vi "Wrist main.vi"() -> ()   [LabVIEW 2018]
uses:
  <vilib>/Rock Robotics/WPI/ThirdParty/Phoenix-LabVIEW/Motor Controller/Controls/CTRE_Phoenix_MotorControl_FeedbackDevice.ctl
  <vilib>/Rock Robotics/WPI/ThirdParty/Phoenix-LabVIEW/Motor Controller/Controls/CTRE_Phoenix_MotorControl_ControlMode.ctl
  <vilib>/Rock Robotics/WPI/ThirdParty/Phoenix-LabVIEW/Motor Controller/Get/CTRE_Phoenix_MotorController_GetSelectedSensorData.vi
panel:
  in  "reset pos":bool
  out "Wrist at home":bool
  in  "Disable?":bool
  in  "Wrist Selector":enum16{"Motion Magic", "Manual", "Disable"}(ring)
  in  "Output":dbl(slide) scale=-1.0..1.0
  in  "Setpoint":dbl
  in  "PIDF":T1={"P"=1.5, "I"=0.0005, "D"=0.0, "F"=0.0, "I zone"=0.0}
  out "Velocity (Raw Sensor Units per 100 ms)":i32
  out "Position (Raw Sensor Units)":i32
  in  "Acceleration":i32
  in  "Cruise Velocity":i32
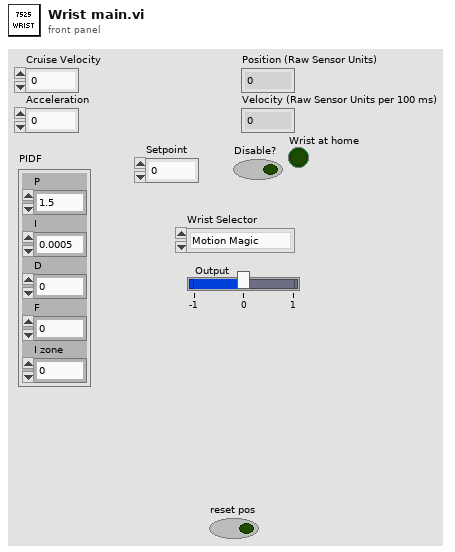
[diagram p1: front panel]
types:
  T1 = cluster{"P":dbl, "I":dbl, "D":dbl, "F":dbl, "I zone":dbl}
  T2 = typedef "CTRE_Phoenix_MotorControl_FeedbackDevice.ctl" = i8
  T3 = typedef "WPI_MotorControlDeviceRef.ctl" = cluster{"DeviceStatus":errorcluster, "Type":T4, "PWM":cluster{"PWM Channel":T5, "DeadBand":T6}, "CAN":cluster{"Device Number":u8, "SetOutput VI Ref":variant, "GetOutput VI Ref":variant, "Enable VI Ref":variant, "Disable VI Ref":variant, "Data":variant}, "Invert":bool, "DIO PWM":cluster{"PWM \"Enable\" Channel":T5, "DIOChannel":T7, "PWM Rate":dbl}}
  T4 = typedef "WPI_MotorControlType.ctl" = enum16{"PWM", "CAN", "DIO PWM"}
  T5 = typedef "FPGA_DIOPWMChannel.ctl" = enum8{"PWM 0", "PWM 1", "PWM 2", "PWM 3", "PWM 4", "PWM 5", "PWM 6", "PWM 7", "PWM 8", "PWM 9", "PWM MXP 0", "PWM MXP 1", "PWM MXP 2", "PWM MXP 3", "PWM MXP 4", "PWM MXP 5", "PWM MXP 6", "PWM MXP 7", "PWM MXP 8", "PWM MXP 9", "Invalid"}
  T6 = typedef "WPI_PWMDeadband.ctl" = cluster{"Name":string, "maxPositivePwm":i32, "minPositivePwm":i32, "centerPwm":i32, "maxNegativePwm":i32, "minNegativePwm":i32, "angularRange":u16}
  T7 = typedef "FPGA_DIOChannel.ctl" = enum8{"DIO 0", "DIO 1", "DIO 2", "DIO 3", "DIO 4", "DIO 5", "DIO 6", "DIO 7", "DIO 8", "DIO 9", "DIO MXP 0", "DIO MXP 1", "DIO MXP 2", "DIO MXP 3", "DIO MXP 4", "DIO MXP 5", "DIO MXP 6", "DIO MXP 7", "DIO MXP 8", "DIO MXP 9", "DIO MXP 10", "DIO MXP 11", "DIO MXP 12", "DIO MXP 13", "DIO MXP 14", "DIO MXP 15", "SPI Port CS1", "SPI Port CS2", "SPI Port CS3", "SPI Port MISO", "SPI Port MOSI", "Invalid"}
  T8 = typedef "CTRE_Phoenix_MotorControl_ControlMode.ctl" = u16
  T9 = typedef "WPI_SwitchDevRef.ctl" = cluster{"DevStatus":errorcluster, "DIO Channel":T7, "CntIndex":T10, "Normally Closed":bool}
  T10 = typedef "FPGA_CounterCtrSystemIndex.ctl" = enum8{"Ctr 0", "Ctr 1", "Ctr 2", "Ctr 3", "Ctr 4", "Ctr 5", "Ctr 6", "Ctr 7", "Invalid"}
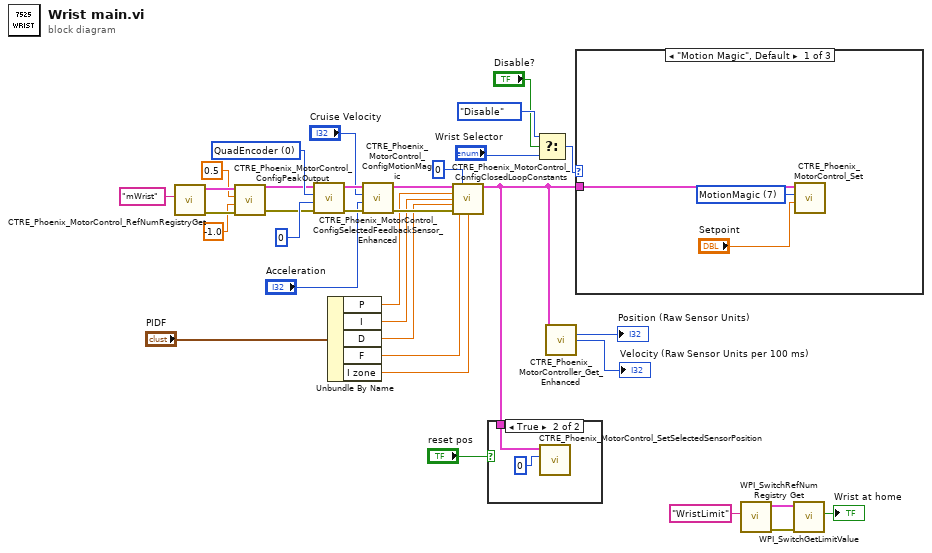
[diagram p0: block diagram]
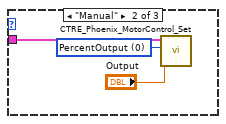
[diagram p3: hidden frame]
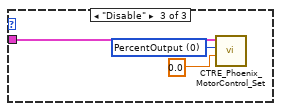
[diagram p4: hidden frame]
diagram:
  w29 = T2 0 items=["QuadEncoder"=0, "Analog"=2, "Tachometer"=4, "Pulse Width Encoded Position"=8, "Sensor Sum (S0 + S1)"=9, "Sensor Difference (D0 - D1)"=10, "Remote Source 0"=11, "Remote Source 1"=12, "Software Emulated"=15] ("Feedback Device")
  n1 = call <vilib>:"CTRE_Phoenix_MotorControl_RefNumRegistryGet.vi"("refnum name"="mWrist") -> ("error out"=w33:errorcluster, "PhoenixMotorControlDevRef"=w32:T3)  [unwired: 9 in]
  n2 = call <vilib>:"CTRE_Phoenix_MotorControl_ConfigPeakOutput.vi"("error in (no error)"=w33, "Reverse Peak Percent Output"=-1.0, "Forward Peak Percent Output"=0.5, "PhoenixMotorControlDevRef"=w32) -> ("error out"=w26:errorcluster, "PhoenixMotorControlDevRef"=w27:T3)  [unwired: 6 in]
  n3 = call <vilib>:"CTRE_Phoenix_MotorControl_ConfigSelectedFeedbackSensor_Enhanced.vi"("error in (no error)"=w26, "pidLoopIdx"=0, "Feedback Device"=w29, "PhoenixMotorControlDevRef"=w27) -> ("error out"=w25:errorcluster, "PhoenixMotorControlDevRef"=w24:T3)  [unwired: 6 in]
  n4 = Unbundle By Name("PIDF") -> ("P"=w15:dbl, "I"=w14:dbl, "D"=w13:dbl, "F"=w12:dbl, "I zone"=w11:dbl)
  n5 = call <vilib>:"CTRE_Phoenix_MotorControl_ConfigMotionMagic.vi"("error in (no error)"=w25, "Acceleration"="Acceleration", "Cruise Velocity"="Cruise Velocity", "PhoenixMotorControlDevRef"=w24) -> ("error out"=w18:errorcluster, "PhoenixMotorControlDevRef"=w19:T3)  [unwired: 6 in]
  n6 = call <vilib>:"CTRE_Phoenix_MotorControl_ConfigClosedLoopConstants.vi"("PhoenixMotorControlDevRef"=w19, "slotIdx"=0, "P"=w15, "I"=w14, "D"=w13, "error in (no error)"=w18, "F"=w12, "I Zone"=w11) -> ("PhoenixMotorControlDevRef"=w1:T3)  [unwired: 6 in, 1 out]
  n7 = case shown="True" "reset pos" {
    tunnel: w1 -> [_ w36]
    frame False {
    }
    frame True {
      n8 = call <vilib>:"CTRE_Phoenix_MotorControl_SetSelectedSensorPosition.vi"("New Sensor Position"=0, "PhoenixMotorControlDevRef"=w36) -> ()  [unwired: 8 in, 2 out]
    }
  }
  n9 = Select(t=enum16{"Motion Magic", "Manual", "Disable"}."Disable", s="Disable?", f="Wrist Selector") -> (s? t:f=w9:enum16{"Motion Magic", "Manual", "Disable"})
  n10 = call-poly <vilib>:"CTRE_Phoenix_MotorController_Get_Enhanced.vi"("PhoenixMotorControlDevRef"=w1) -> ("Position (Raw Sensor Units)"=→"Position (Raw Sensor Units)":i32, "Velocity (Raw Sensor Units per 100 ms)"=→"Velocity (Raw Sensor Units per 100 ms)":i32)  [unwired: 11 in, 2 out]
  n11 = case shown="\"Motion Magic\", Default" w9 {
    tunnel: w1 -> [w38 w42 w44]
    frame "Motion Magic", Default {
      w39 = T8 7 items=["PercentOutput"=0, "Position"=1, "Velocity"=2, "Current"=3, "Follower"=5, "MotionProfile"=6, "MotionMagic"=7, "MotionProfileArc"=10, "Disabled"=15] ("Control Mode")
      n12 = call <vilib>:"CTRE_Phoenix_MotorControl_Set.vi"("Output"="Setpoint", "Control Mode"=w39, "PhoenixMotorControlDevRef"=w38) -> ()  [unwired: 7 in, 2 out]
    }
    frame "Manual" {
      w41 = T8 0 items=["PercentOutput"=0, "Position"=1, "Velocity"=2, "Current"=3, "Follower"=5, "MotionProfile"=6, "MotionMagic"=7, "MotionProfileArc"=10, "Disabled"=15] ("Control Mode")
      n13 = call <vilib>:"CTRE_Phoenix_MotorControl_Set.vi"("Output"="Output", "Control Mode"=w41, "PhoenixMotorControlDevRef"=w42) -> ()  [unwired: 7 in, 2 out]
    }
    frame "Disable" {
      w45 = T8 0 items=["PercentOutput"=0, "Position"=1, "Velocity"=2, "Current"=3, "Follower"=5, "MotionProfile"=6, "MotionMagic"=7, "MotionProfileArc"=10, "Disabled"=15] ("Control Mode")
      n14 = call <vilib>:"CTRE_Phoenix_MotorControl_Set.vi"("Output"=0.0, "Control Mode"=w45, "PhoenixMotorControlDevRef"=w44) -> ()  [unwired: 7 in, 2 out]
    }
  }
  n15 = call <vilib>:"WPI_SwitchRefNum Registry Get.vi"("refnum name"="WristLimit") -> ("error out"=w6:errorcluster, "SwitchDevRef"=w5:T9)  [unwired: 9 in]
  n16 = call <vilib>:"WPI_SwitchGetLimitValue.vi"("error in (no error)"=w6, "SwitchDevRef"=w5) -> ("Switch Pressed"=→"Wrist at home":bool)  [unwired: 7 in, 2 out]
